vi "Spreadsheet String to Array.vi"() -> ()   [LabVIEW 2016, in "User Interface.lvlib"]
uses:
  User Interface.lvlib
panel:
  in  "String input":string
  out "array":string[](array[string])
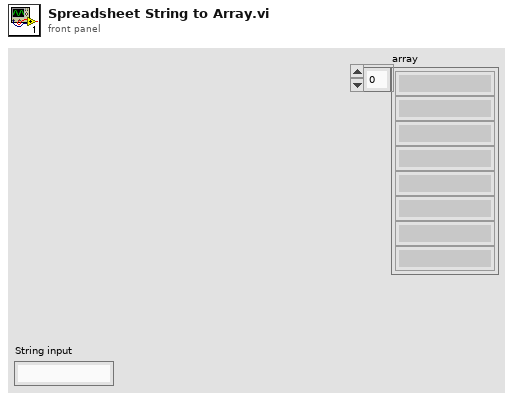
[diagram p1: front panel]
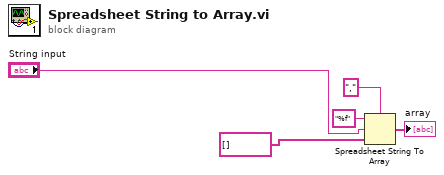
[diagram p0: block diagram]
diagram:
  n1 = Spreadsheet String To Array(delimiter (Tab)=",", format string="%f", spreadsheet string="String input", array type (2D Dbl)=string[] []) -> (array=→"array":string[])
